vi "bit2ASII.vi"(9 "message_bit":i8[](array[numeric]), 10 "code":enum16{"无编码", "RS码", "卷积码"}(ring)) -> (2 "数据字符串 2":string)   [LabVIEW 2010]
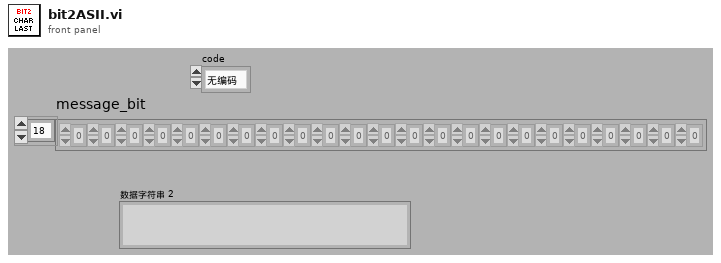
[diagram p1: front panel]
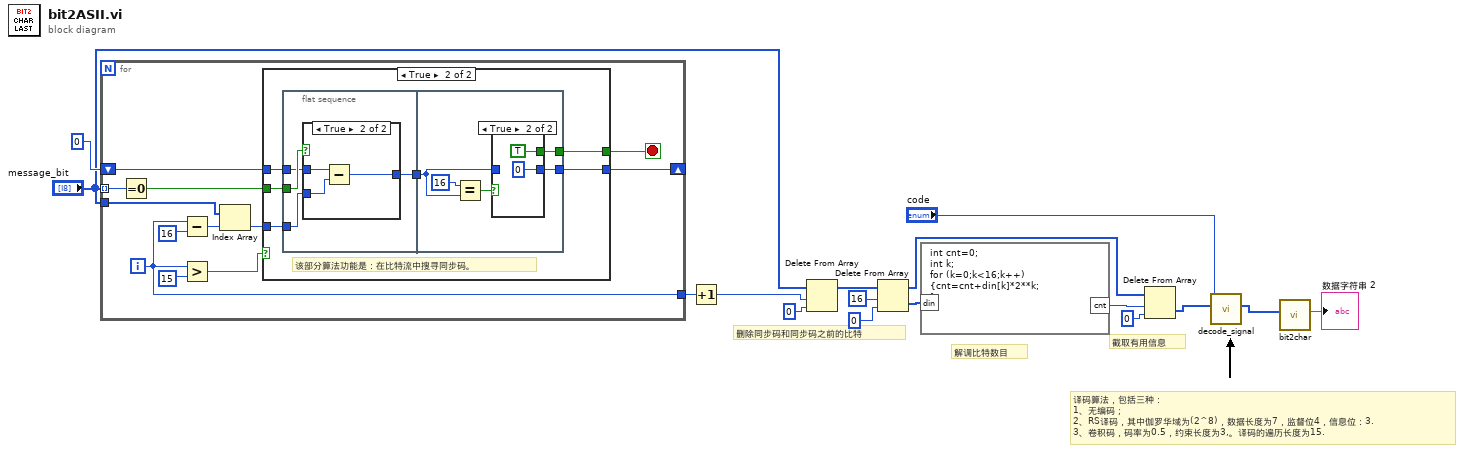
[diagram p0: block diagram]
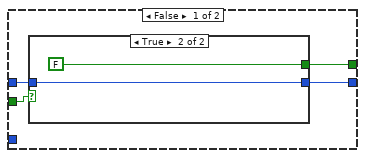
[diagram p2: hidden frame]
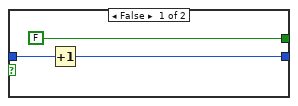
[diagram p3: hidden frame]
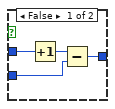
[diagram p4: hidden frame]
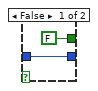
[diagram p5: hidden frame]
diagram:
  # "译码算法，包括三种：\n1、无编码；\n2、RS译码，其中伽罗华域为(2^8)，数据长度为7，监督位4，信息位：3.\n3、卷积码，码率为0.5，约束长度为3,。译码的遍历长度为15."
  # "截取有用信息"
  # "解调比特数目"
  # "删除同步码和同步码之前的比特"
  n1 = for {
    tunnel: "message_bit" -> [w28] mode=indexing
    shift-right: [w23] -> _
    shift-left: 0 -> [w27]
    tunnel: "message_bit" -> [w26]
    tunnel: [w17] -> w15
    i -> [w17]
    stop <- w18 stop-if-true
    n2 = Equal To 0?(x=w28) -> (x = 0?=w24:bool)
    n3 = Subtract(x=w17, y=16) -> (x-y=w20:i32)
    n4 = Greater?(x=w17, y=15) -> (0:w22:bool)
    n5 = Index Array(array=w26, index=w20) -> (element=w19:i8)
    n6 = case shown="True" w22 {
      tunnel: w27 -> [w31 w41]
      tunnel: w24 -> [w32 w43]
      tunnel: [w30 w38] -> w23
      tunnel: w19 -> [_ w42]
      tunnel: [w29 w39] -> w18
      frame False {
        n7 = case shown="True" w32 {
          tunnel: w31 -> [w35 w37]
          tunnel: [w34 w37] -> w30
          tunnel: [FALSE FALSE] -> w29
          frame False {
            n8 = Increment(x=w35) -> (x+1=w34:i32)
          }
          frame True {
          }
        }
      }
      frame True {
        # "该部分算法功能是：在比特流中搜寻同步码。"
        n9 = flat-sequence {
          tunnel: w43 -> [w47]
          tunnel: w42 -> [w46]
          tunnel: w41 -> [w45]
          tunnel: [w44] -> w40
          tunnel: w40 -> [w55]
          tunnel: [w57] -> w39
          tunnel: [w56] -> w38
          frame #0 {
            n10 = case shown="True" w47 {
              tunnel: w46 -> [w49 w54]
              tunnel: w45 -> [w51 w53]
              tunnel: [w48 w52] -> w44
              frame False {
                n11 = Increment(x=w51) -> (x+1=w50:i32)
                n12 = Subtract(x=w50, y=w49) -> (x-y=w48:i32)
              }
              frame True {
                n13 = Subtract(x=w53, y=w54) -> (x-y=w52:i32)
              }
            }
          }
          frame #1 {
            n14 = Equal?(x=16, y=w55) -> (x = y?=w58:bool)
            n15 = case shown="True" w58 {
              tunnel: [FALSE TRUE] -> w57
              tunnel: [w61 0] -> w56
              tunnel: w55 -> [w61 _]
              frame False {
              }
              frame True {
              }
            }
          }
        }
      }
    }
  }
  n16 = Increment(x=w15) -> (x+1=w1:i32)
  n17 = Delete From Array(array="message_bit", length=w1, index=0 ("索引")) -> (array with subset deleted=w13:i8[])  [unwired: 1 out]
  n18 = Delete From Array(array=w13, length=16 ("长度"), index=0 ("索引")) -> (deleted portion=w10:i8[], array with subset deleted=w7:i8[])
  n19 = formula code="int cnt=0;\nint k;\nfor (k=0;k<16;k++)\n{cnt=cnt+din[k]*2**k;\n}"("din"=w10) -> ("cnt"=w9:i32)
  n20 = Delete From Array(array=w7, length=w9, index=0 ("索引")) -> (deleted portion=w4:i8[])  [unwired: 1 out]
  n21 = call "decode_signal.vi"("signal_in"=w4, "code"="code") -> ("decode_symbol"=w3:i8[])  [unwired: 8 in, 1 out]
  n22 = call "bit2char.vi"("input bit stream"=w3) -> ("数据字符串 2"=→"数据字符串 2":string)  [unwired: 10 in]
